vi "rbw.vi"(8 "Error in":errorcluster, 10 "RBW (kHz)":u32=300, 11 "VISA name in":refnum<visa-resource-name>) -> (0 "Error out":errorcluster, 3 "VISA name out":refnum<visa-resource-name>)   [LabVIEW 2012]
panel:
  out "cmd terminate":string
  out "cmd echo":string
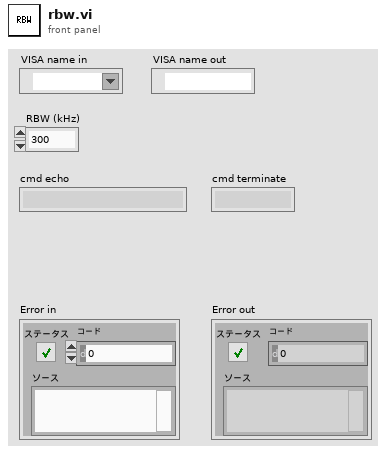
[diagram p1: front panel]
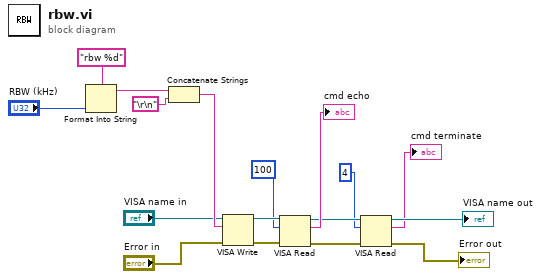
[diagram p0: block diagram]
diagram:
  n1 = Format Into String(format string="rbw %d" ("形式文字列"), "RBW (kHz)") -> (resulting string=w9:string)  [unwired: 2 in, 1 out]
  n2 = Concatenate Strings(w9, "\r\n") -> (w16:string)
  n3 = VISA Write(VISA resource name="VISA name in", write buffer=w16, error in (no error)="Error in") -> (VISA resource name out=w14:refnum<visa-resource-name>, error out=w13:errorcluster)  [unwired: 1 out]
  n4 = VISA Read(VISA resource name=w14, byte count=u32 100 ("バイトカウント"), error in (no error)=w13) -> (VISA resource name out=w6:refnum<visa-resource-name>, read buffer=→"cmd echo":string, error out=w4:errorcluster)  [unwired: 1 out]
  n5 = VISA Read(VISA resource name=w6, byte count=u32 4 ("バイトカウント"), error in (no error)=w4) -> (VISA resource name out=→"VISA name out":refnum<visa-resource-name>, read buffer=→"cmd terminate":string, error out=→"Error out":errorcluster)  [unwired: 1 out]
